vi "checkRight.vi"(8 "错误输入（无错误）":errorcluster) -> (0 "错误输出":errorcluster, 3 "是否合法":bool)   [LabVIEW 2014]
uses:
  kernel32.dll
panel:
  out "return type":string
  out "数值":i32=12
  out "硬盘序列号":string
  out "数值 3":i32=12
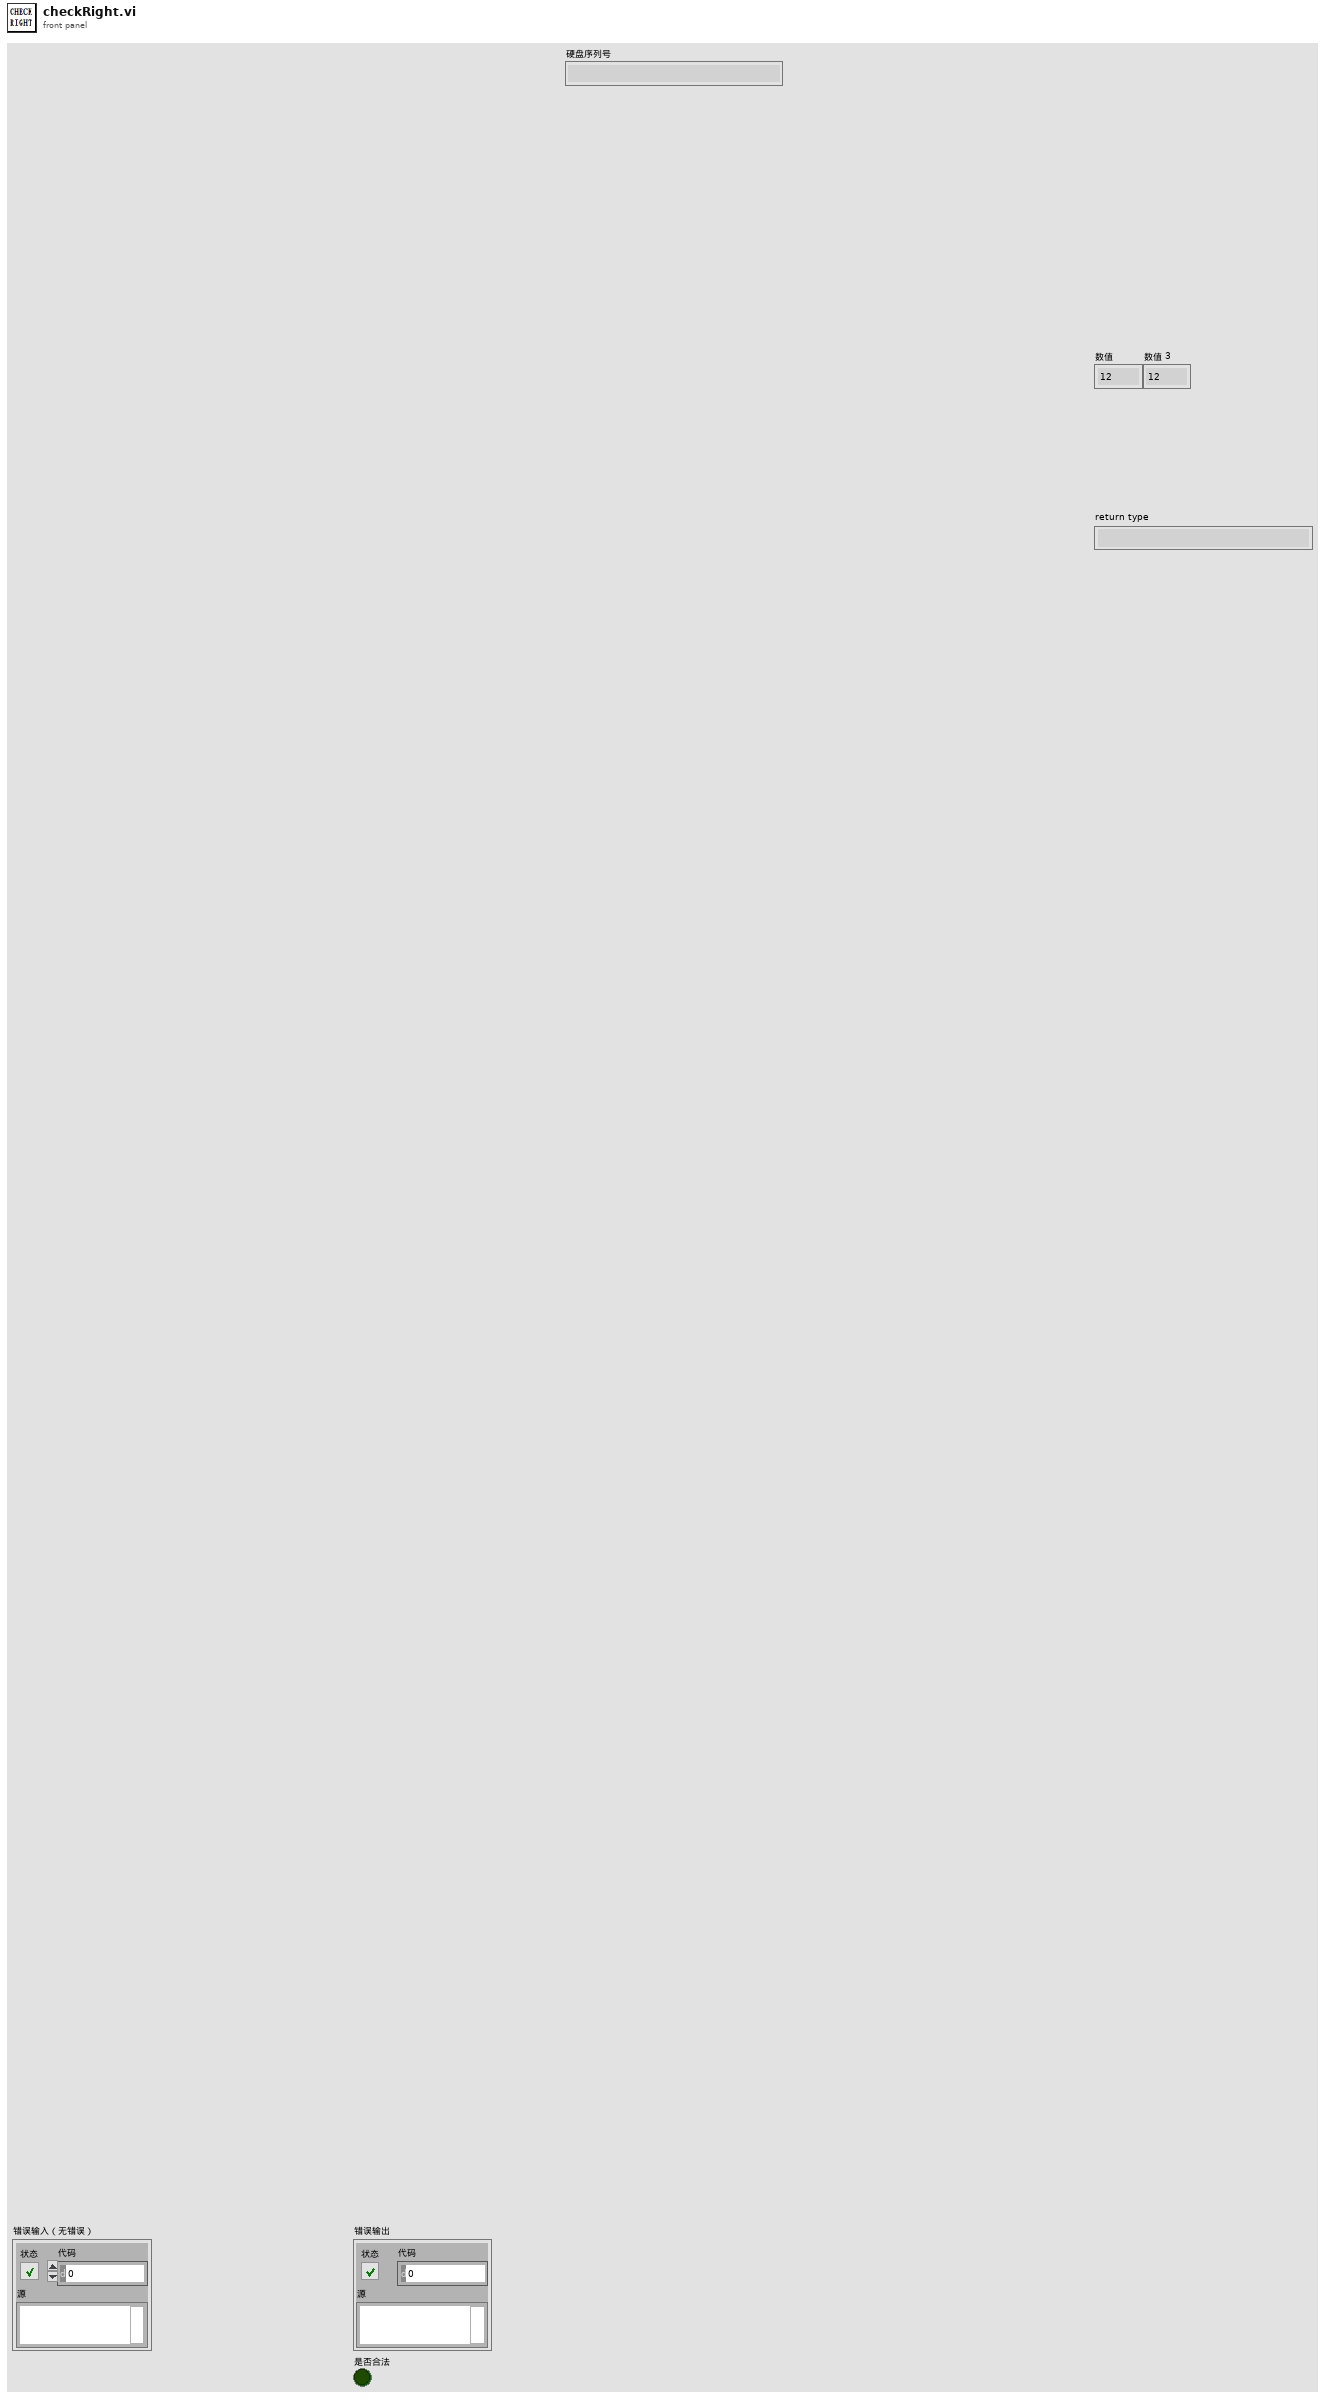
[diagram p1: front panel]
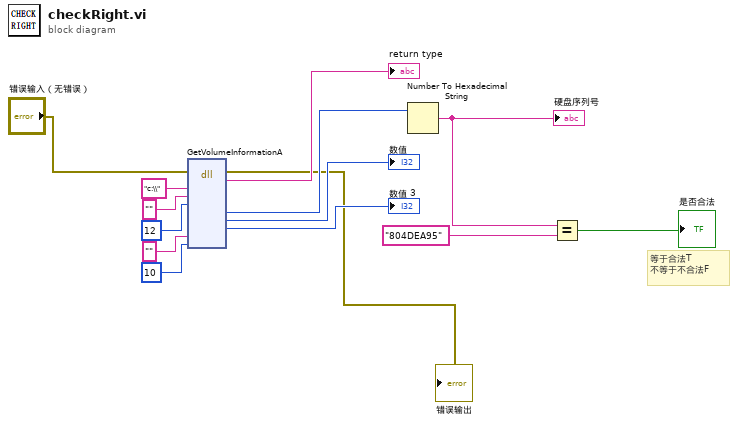
[diagram p0: block diagram]
diagram:
  # "等于合法T\n不等于不合法F"
  n1 = dll-call lib="kernel32.dll" fn="GetVolumeInformationA"(error in="错误输入（无错误）", "lpRootPathName"="c:\\", "lpRootPathName"="", "nVolumeNameSize"=12, "lpFileSystemNameBuffer"="", "nFileSystemNameSize"=10) -> (error out=→"错误输出":errorcluster, "return type"=→"return type":string, "VolumeSerialNumber"=w10:i32, "MaximumComponentLength"=→"数值":i32, "FileSystemFlags"=→"数值 3":i32)  [unwired: 10 in, 1 out]
  n2 = Number To Hexadecimal String(2:w10) -> (0:w13:string)  [unwired: 1 in]
  "硬盘序列号" <- w13
  n3 = Equal?(x=w13, y="804DEA95") -> (x = y?=→"是否合法":bool)
